vi "Write Channels_ Lockin.vi"(8 "error in (no error)":errorcluster, 10 "Channels: Lockin":T1={"REF f (Hz)"=[13.0], "REF phi (°)"=[0.0, 0.0, 0.0, 0.0, 0.0, 0.0, 0.0, 0.0]} {"REF phi (°)" format="%#_3g"}, 11 "Instrument.Lockin in":refnum<class "Instrument.Lockin.lvclass">) -> (0 "error out":errorcluster, 3 "Instrument.Lockin out":refnum<class "Instrument.Lockin.lvclass">)   [LabVIEW 2016, in "Instrument.Lockin.lvclass"]
uses:
  Instrument.Lockin.lvclass
  Typedefs/REF-cluster.ctl
  Typedefs/REF_f-array.ctl
  Typedefs/REF_phi-array.ctl
  Instrument.Lockin.lvclass/Instrument.Lockin.ctl
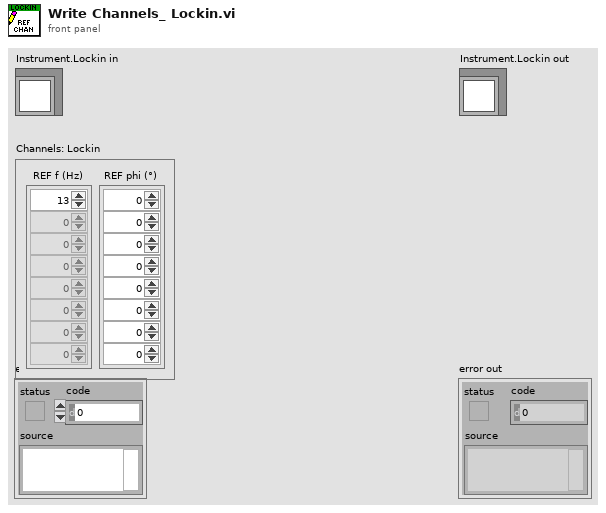
[diagram p1: front panel]
types:
  T1 = typedef "Instrument.Lockin.lvclass/REF-cluster.ctl" = cluster{"REF f (Hz)":T2, "REF phi (°)":T3}
  T2 = typedef "Instrument.Lockin.lvclass/REF_f-array.ctl" = dbl[]
  T3 = typedef "Instrument.Lockin.lvclass/REF_phi-array.ctl" = dbl[]
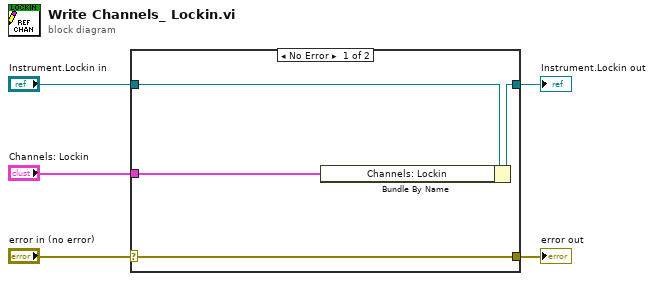
[diagram p0: block diagram]
diagram:
  n1 = case shown="No Error" "error in (no error)" {
    selector: "error in (no error)" -> [w9 w10]
    tunnel: [w9 w10] -> w4
    tunnel: [w7 w11] -> w2
    tunnel: "Instrument.Lockin in" -> [w8 w11]
    tunnel: "Channels: Lockin" -> [w6 _]
    frame No Error {
      n2 = Bundle By Name(cluster=w8, "Channels: Lockin"=w6) -> (w7:refnum<class "Instrument.Lockin.lvclass">)
    }
    frame Error {
    }
  }
  "error out" <- w4
  "Instrument.Lockin out" <- w2
